vi "BlinkELVISDigitalOutsExample.vi"() -> ()   [LabVIEW 2018]
panel:
  in  "Blink\n2":bool
  in  "Blink\n1":bool
  in  "Blink\n0":bool
  out "2":bool
  out "1":bool
  out "0":bool
  in  "Blink Duration (s)":dbl=1.0
  in  "stop":bool
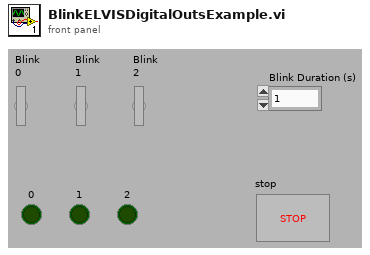
[diagram p1: front panel]
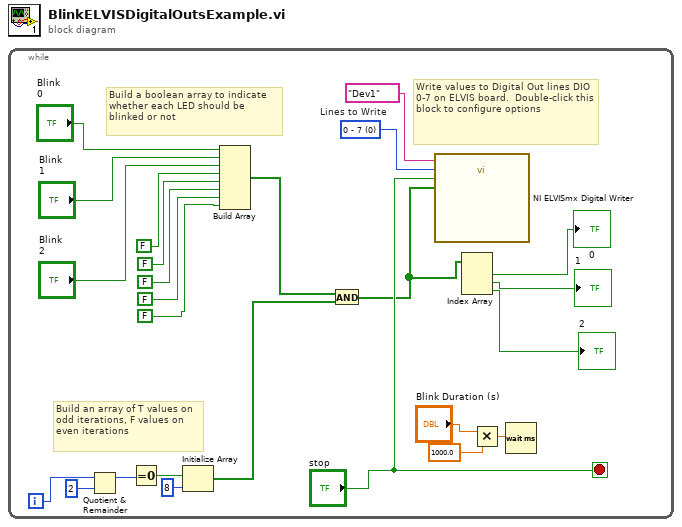
[diagram p0: block diagram]
diagram:
  n1 = while {
    i -> [w12]
    stop <- "stop" stop-if-true
    w24 = u16 0 items=["0 - 7", "8 - 15", "16 - 23"]  # Lines to Write
    # "Write values to Digital Out lines DIO 0-7 on ELVIS board.  Double-click this block to configure options"
    # "Build a boolean array to indicate whether each LED should be blinked or not"
    # "Build an array of T values on odd iterations, F values on even iterations"
    n2 = Quotient & Remainder(x=w12, y=2) -> (x-y*floor(x/y)=w9:i32)  [unwired: 1 out]
    n3 = Equal To 0?(x=w9) -> (x = 0?=w8:bool)
    n4 = Initialize Array(w8, 8 ("dimension size")) -> (w6:bool[])
    n5 = Build Array("Blink\n0", "Blink\n1", "Blink\n2", FALSE, FALSE, FALSE, FALSE, FALSE) -> (w10:bool[])
    n6 = And(x=w10, y=w6) -> (x .and. y?=w5:bool[])
    n7 = call "NI ELVISmx Digital Writer"("Device Name"=tag "Dev1", "Lines to Write"=w24, "Stop"="stop", "DO Lines"=w5) -> ()  [unwired: 15 in, 1 out]
    n8 = Index Array(array=w5) -> (element #1=→"0":bool, element #2=→"1":bool, element #3=→"2":bool)  [unwired: 3 in]
    n9 = Multiply(x="Blink Duration (s)", y=1000.0) -> (x*y=w23:dbl)
    n10 = Wait (ms)(milliseconds to wait=w23) -> ()  [unwired: 1 out]
  }
